vi "SupplyRamp.vi"(6 "error in":errorcluster, 7 "Requested Voltage":dbl format="%.2f", 8 "Step Size":dbl step=1.0 format="%.1f", 9 "Step Delay":u32 step=1, 10 "Supply IN":refnum<class "SupplyControl.lvclass">, 11 "Starting Voltage":dbl format="%.2f") -> (0 "error out":errorcluster, 1 "Supply OUT":refnum<class "SupplyControl.lvclass">, 2 "Compliance exceeded":bool, 3 "Current Voltage":dbl format="%.2f")   [LabVIEW 2018, in "SupplyControl.lvclass"]
uses:
  SupplyControl.lvclass
panel:
  out "requested volts":dbl format="%.1f"
  out "Progress":dbl(slide) min=0.0 max=1.0 scale=0.0..1.0 scale format="%.1f"
  in  "stop":bool
  out "starting volts":dbl format="%.1f"
  # "Voltage Ramp in Progress"
  # "Ramping from"
  # "to"
  # "volts"
  # "in steps of"
  # "volts every"
  # "msec(s)"
  # "Status"
  # "Current Voltage:"
  # "Compliance:"
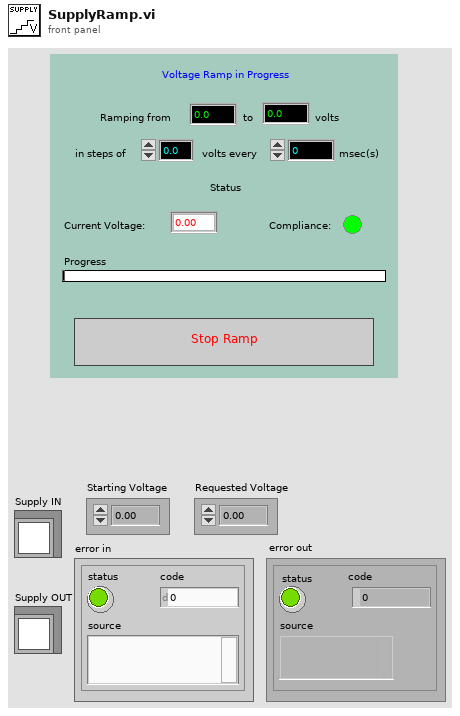
[diagram p1: front panel]
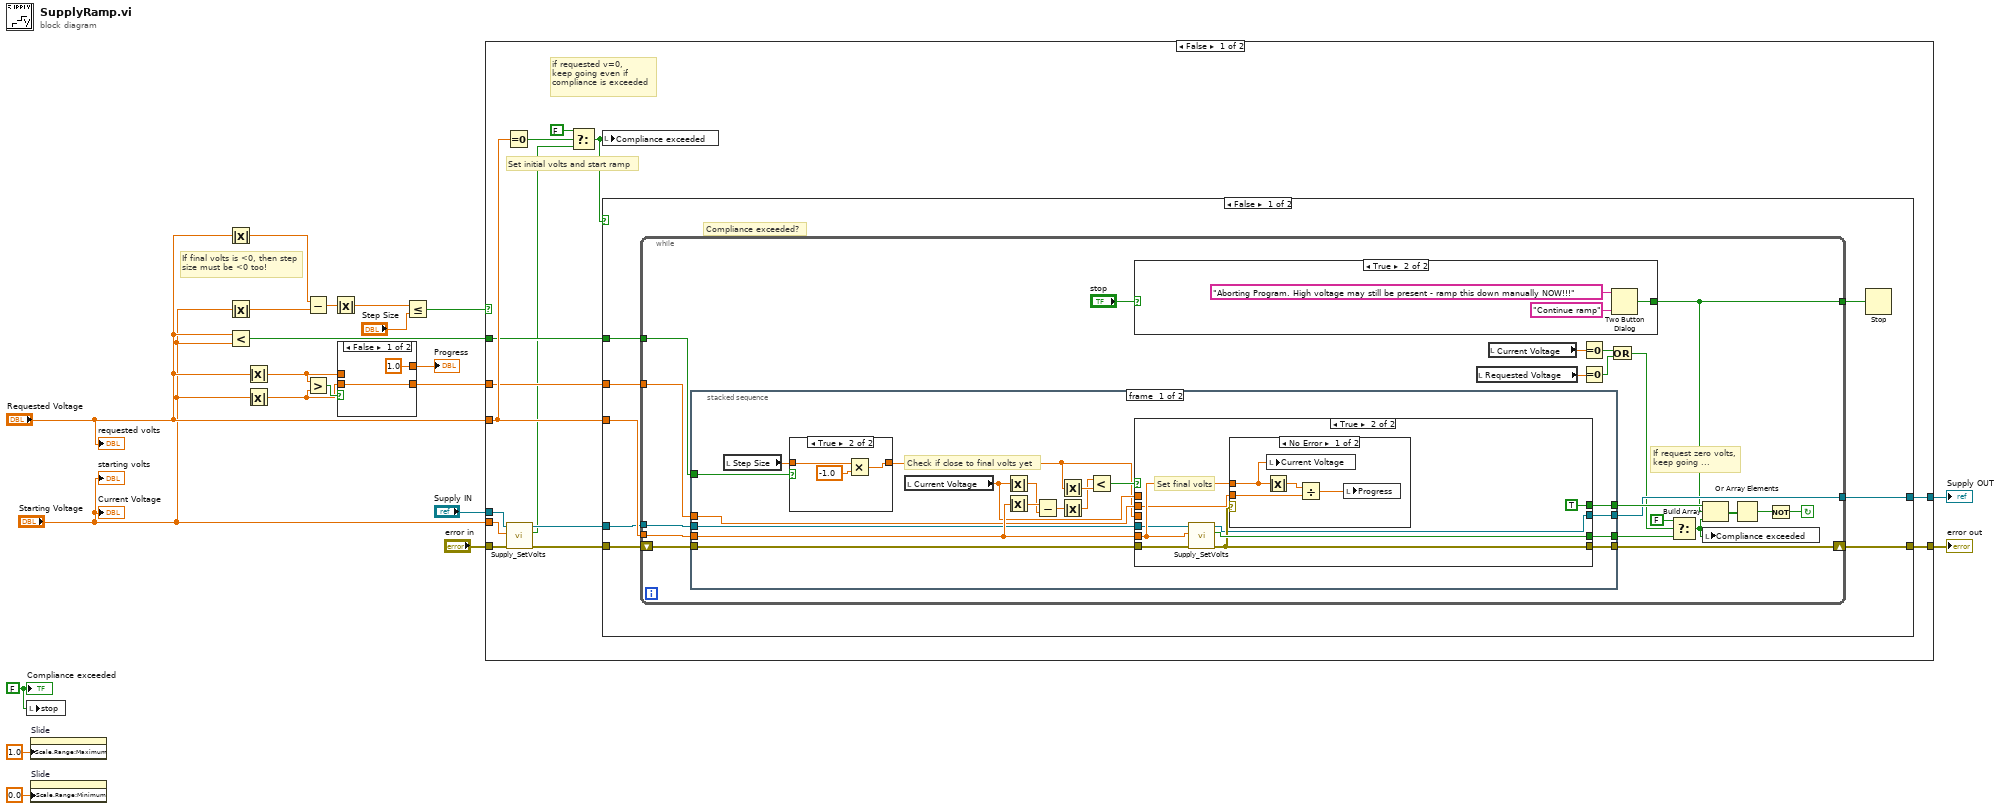
[diagram p0: block diagram]
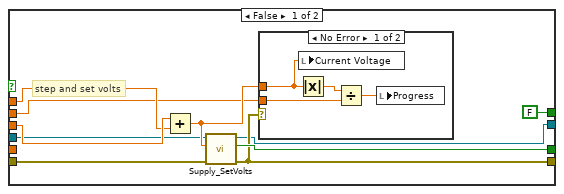
[diagram p4: hidden frame]
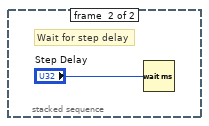
[diagram p7: hidden frame]
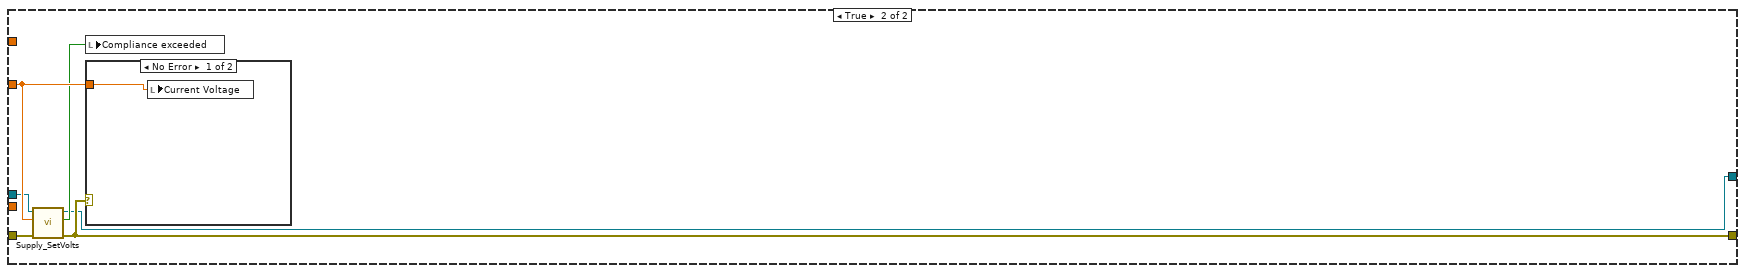
[diagram p9: hidden frame]
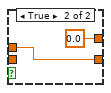
[diagram p11: hidden frame]
diagram:
  w3 = FALSE
  # "If final volts is <0, then step\nsize must be <0 too!"
  n1 = local write "stop"(w3) -> ()
  n2 = property on="Slide" class="Slide (strict)"("Scale.Range:Maximum"=1.0) -> ()  [unwired: 2 in, 2 out]
  n3 = property on="Slide" class="Slide (strict)"("Scale.Range:Minimum"=0.0) -> ()  [unwired: 2 in, 2 out]
  n4 = Absolute Value(x="Requested Voltage") -> (abs(x)=w21:dbl)
  n5 = Absolute Value(x="Starting Voltage") -> (abs(x)=w20:dbl)
  n6 = Less?(x="Requested Voltage", y="Starting Voltage") -> (x < y?=w8:bool)
  n7 = Absolute Value(x="Requested Voltage") -> (abs(x)=w15:dbl)
  n8 = Absolute Value(x="Starting Voltage") -> (abs(x)=w14:dbl)
  n9 = Subtract(x=w21, y=w20) -> (x-y=w18:dbl)
  n10 = Greater?(x=w15, y=w14) -> (0:w16:bool)
  n11 = Absolute Value(x=w18) -> (abs(x)=w17:dbl)
  n12 = case shown="False" w16 {
    tunnel: w15 -> [_ w25]
    tunnel: w14 -> [w23 _]
    tunnel: [w23 w25] -> w13
    tunnel: [1.0 0.0] -> w12
    frame False {
    }
    frame True {
    }
  }
  "Progress" <- w12
  n13 = Less Or Equal?(x=w17, y="Step Size") -> (x <= y?=w19:bool)
  n14 = case shown="False" w19 {
    tunnel: "Starting Voltage" -> [w39 _]
    tunnel: "Requested Voltage" -> [w38 w129]
    tunnel: w13 -> [w37 _]
    tunnel: w8 -> [w36 _]
    tunnel: [w33 w128] -> w5
    tunnel: "error in" -> [w34 w126]
    tunnel: "Supply IN" -> [w32 w125]
    tunnel: [w30 w124] -> w1
    frame False {
      # "if requested v=0,\nkeep going even if\ncompliance is exceeded"
      # "Set initial volts and start ramp"
      n15 = Equal To 0?(x=w38) -> (x = 0?=w29:bool)
      n16 = call-dynamic "Supply_SetVolts.vi"("error in (no error)"=w34, "Volts IN [V]"=w39, "SupplyControl in"=w32) -> ("error out"=w35:errorcluster, "Compliance exceeded?"=w27:bool, "SupplyControl out"=w31:refnum<class "SupplyControl.lvclass">)  [unwired: 6 in]
      n17 = Select(t=FALSE, s=w29, f=w27) -> (s? t:f=w26:bool)
      n18 = local write "Compliance exceeded"(w26) -> ()
      n19 = case shown="False" w26 {
        tunnel: w35 -> [w44 w123]
        tunnel: w38 -> [w47 _]
        tunnel: w37 -> [w46 _]
        tunnel: w36 -> [w45 _]
        tunnel: [w43 w123] -> w33
        tunnel: w31 -> [w42 w122]
        tunnel: [w41 w122] -> w30
        frame False {
          # "Compliance exceeded?"
          n20 = while {
            tunnel: w45 -> [w61]
            tunnel: w46 -> [w62]
            tunnel: w47 -> [w68]
            shift-right: [w56] -> w43
            shift-left: w44 -> [w55]
            tunnel: w42 -> [w54]
            tunnel: [w53] -> w41
            tunnel: [w52] -> w40
            stop <- w65 continue-if-true
            # "If request zero volts,\nkeep going ..."
            n21 = stacked-sequence {
              tunnel: w68 -> [w85 _]
              tunnel: [w86 _] -> w67
              tunnel: w55 -> [w76 _]
              tunnel: [w83 _] -> w48
              tunnel: w62 -> [w80 _]
              tunnel: w61 -> [w78 _]
              tunnel: [w75 _] -> w56
              tunnel: w54 -> [w74 _]
              tunnel: [w73 _] -> w53
              frame #0 {
                # "Check if close to final volts yet"
                n22 = local read "Step Size"() -> (w79:dbl)
                n23 = case shown="True" w78 {
                  tunnel: w79 -> [w91 w94]
                  tunnel: [w91 w92] -> w77
                  frame False {
                  }
                  frame True {
                    n24 = Multiply(x=w94, y=-1.0) -> (x*y=w92:dbl)
                  }
                }
                n25 = local read "Current Voltage"() -> (w84:dbl)
                n26 = Absolute Value(x=w84) -> (abs(x)=w89:dbl)
                n27 = Absolute Value(x=w85) -> (abs(x)=w90:dbl)
                n28 = Subtract(x=w90, y=w89) -> (x-y=w82:dbl)
                n29 = Absolute Value(x=w77) -> (abs(x)=w88:dbl)
                n30 = Absolute Value(x=w82) -> (abs(x)=w81:dbl)
                n31 = Less?(x=w81, y=w88) -> (x < y?=w87:bool)
                n32 = case shown="True" w87 {
                  tunnel: w84 -> [w103 _]
                  tunnel: w77 -> [w104 _]
                  tunnel: [FALSE TRUE] -> w86
                  tunnel: w85 -> [_ w115]
                  tunnel: [w99 w114] -> w83
                  tunnel: w80 -> [w100 w113]
                  tunnel: w76 -> [w98 w112]
                  tunnel: [w97 w111] -> w75
                  tunnel: w74 -> [w96 w110]
                  tunnel: [w95 w109] -> w73
                  frame False {
                    # "step and set volts"
                    n33 = Add(x=w104, y=w103) -> (x+y=w101:dbl)
                    n34 = call-dynamic "Supply_SetVolts.vi"("error in (no error)"=w98, "Volts IN [V]"=w101, "SupplyControl in"=w96) -> ("error out"=w97:errorcluster, "Compliance exceeded?"=w99:bool, "SupplyControl out"=w95:refnum<class "SupplyControl.lvclass">)  [unwired: 6 in]
                    n35 = case shown="No Error" w97 {
                      tunnel: w101 -> [w105 _]
                      tunnel: w100 -> [w107 _]
                      frame No Error {
                        n36 = Absolute Value(x=w105) -> (abs(x)=w108:dbl)
                        n37 = local write "Current Voltage"(w105) -> ()
                        n38 = Divide(x=w108, y=w107) -> (x/y=w106:dbl)
                        n39 = local write "Progress"(w106) -> ()
                      }
                      frame Error {
                      }
                    }
                  }
                  frame True {
                    # "Set final volts"
                    n40 = call-dynamic "Supply_SetVolts.vi"("error in (no error)"=w112, "Volts IN [V]"=w115, "SupplyControl in"=w110) -> ("error out"=w111:errorcluster, "Compliance exceeded?"=w114:bool, "SupplyControl out"=w109:refnum<class "SupplyControl.lvclass">)  [unwired: 6 in]
                    n41 = case shown="No Error" w111 {
                      tunnel: w115 -> [w120 _]
                      tunnel: w113 -> [w118 _]
                      frame No Error {
                        n42 = Absolute Value(x=w120) -> (abs(x)=w119:dbl)
                        n43 = local write "Current Voltage"(w120) -> ()
                        n44 = Divide(x=w119, y=w118) -> (x/y=w117:dbl)
                        n45 = local write "Progress"(w117) -> ()
                      }
                      frame Error {
                      }
                    }
                  }
                }
              }
              frame #1 {
                # "Wait for step delay"
                n46 = Wait (ms)(milliseconds to wait="Step Delay") -> ()  [unwired: 1 out]
              }
            }
            n47 = case shown="True" "stop" {
              selector: "stop" -> [w69 _]
              tunnel: [w69 w72] -> w52
              frame False {
              }
              frame True {
                n48 = Two Button Dialog(message="Aborting Program. High voltage may still be present - ramp this down manually NOW!!!", 1:"Continue ramp" ("F button name (\"Cancel\")")) -> (T button?=w72:bool)  [unwired: 1 in]
              }
            }
            n49 = local read "Requested Voltage"() -> (w63:dbl)
            n50 = local read "Current Voltage"() -> (w57:dbl)
            n51 = Equal To 0?(x=w57) -> (x = 0?=w58:bool)
            n52 = Equal To 0?(x=w63) -> (x = 0?=w59:bool)
            n53 = Or(x=w58, y=w59) -> (x .or. y?=w51:bool)
            n54 = Select(t=FALSE, s=w51, f=w48) -> (s? t:f=w49:bool)
            n55 = Build Array(w67, w52, w49) -> (w64:bool[])
            n56 = local write "Compliance exceeded"(w49) -> ()
            n57 = Or Array Elements(Boolean array=w64) -> (logical OR=w66:bool)
            n58 = Not(x=w66) -> (.not. x?=w65:bool)
          }
          n59 = Stop(stop? (T)=w40) -> ()
        }
        frame True {
          # "Compliance exceeded on initial step"
        }
      }
    }
    frame True {
      n60 = call-dynamic "Supply_SetVolts.vi"("error in (no error)"=w126, "Volts IN [V]"=w129, "SupplyControl in"=w125) -> ("error out"=w128:errorcluster, "Compliance exceeded?"=w127:bool, "SupplyControl out"=w124:refnum<class "SupplyControl.lvclass">)  [unwired: 6 in]
      n61 = local write "Compliance exceeded"(w127) -> ()
      n62 = case shown="No Error" w128 {
        tunnel: w129 -> [w130 _]
        frame No Error {
          n63 = local write "Current Voltage"(w130) -> ()
        }
        frame Error {
        }
      }
    }
  }
  "error out" <- w5
  "Supply OUT" <- w1
  "Current Voltage" <- "Starting Voltage"
  "starting volts" <- "Starting Voltage"
  "requested volts" <- "Requested Voltage"
  "Compliance exceeded" <- w3
